vi "Clear Filter Wheel Timeout Flag.vi"(0 "Session Handle in":T1, 11 "error in (no error)":errorcluster) -> (4 "Session Handle out":T1, 6 "Success?":bool, 8 "Error Code":string, 15 "error out":errorcluster)   [LabVIEW 2015, in "PAS.lvclass"]
uses:
  PAS.lvclass
  Typedefs/Session Handle.ctl
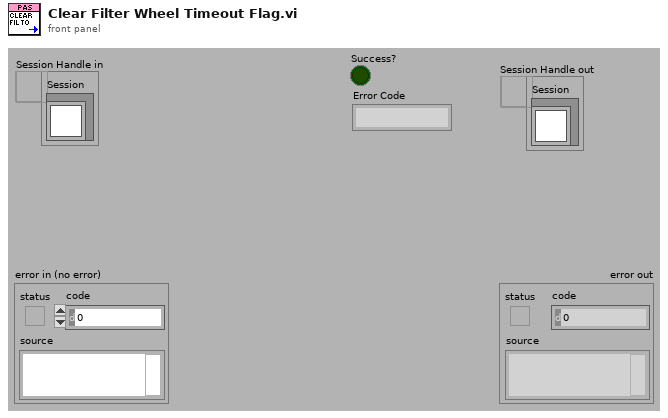
[diagram p1: front panel]
types:
  T1 = typedef "PAS.lvclass/Session Handle.ctl" = refnum<data-value>
  T2 = typedef "XNET Frame CAN.ctl" = cluster{"timestamp":timestamp, "payload":u8[], "identifier":u32, "type":T3, "extended?":bool, "echo?":bool}
  T3 = typedef "XNET Frame Type CAN.ctl" = u8
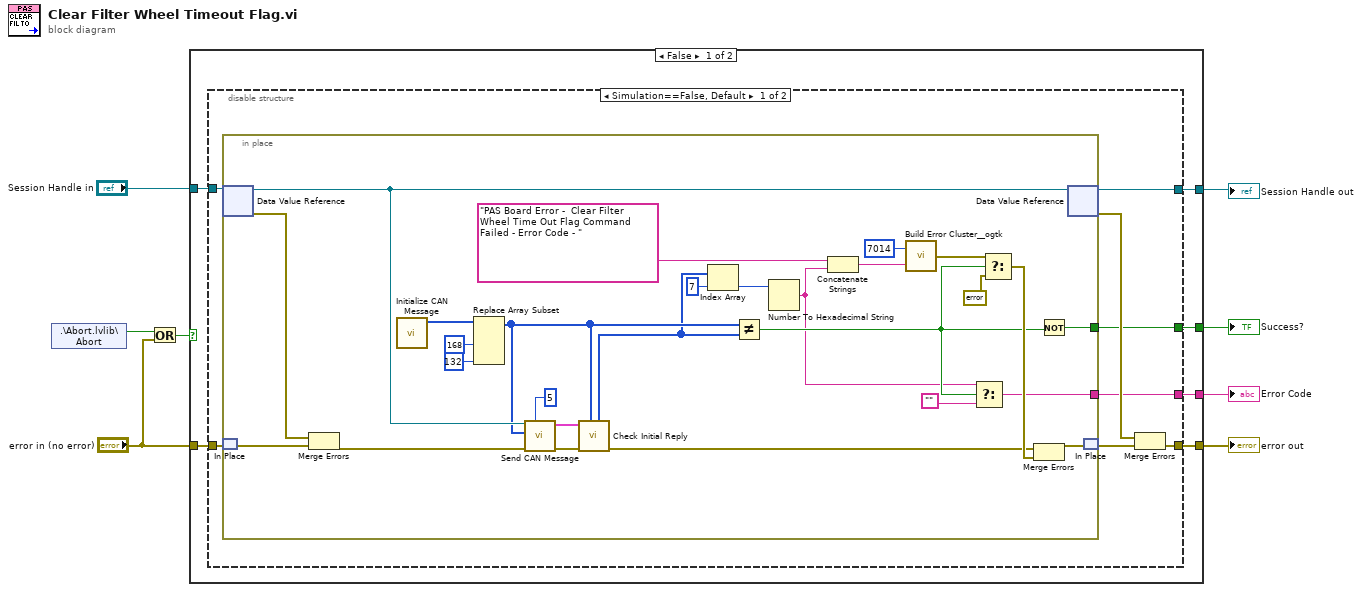
[diagram p0: block diagram]
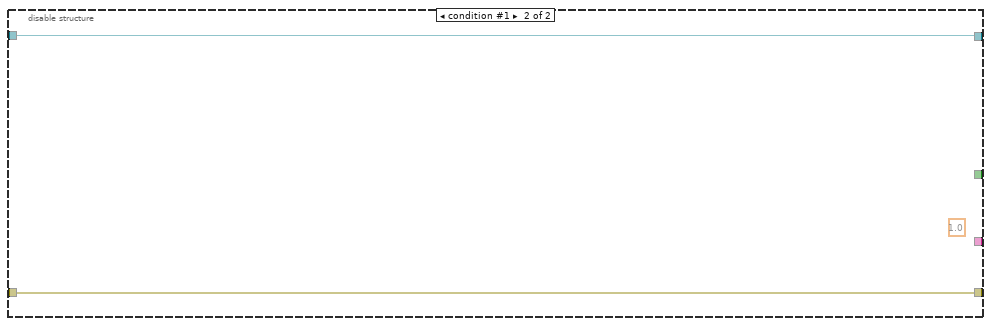
[diagram p2: hidden frame]
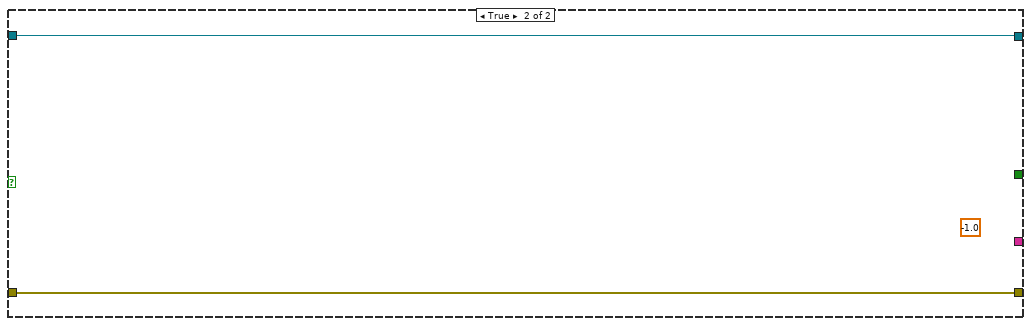
[diagram p3: hidden frame]
diagram:
  n1 = shared-variable ".\\Abort.lvlib\\Abort"() -> (w5:bool)  [unwired: 1 in, 1 out]
  n2 = Or(x=w5, y="error in (no error)") -> (x .or. y?=w3:bool)
  n3 = case shown="False" w3 {
    tunnel: [w14 w53] -> w7
    tunnel: [w13 w52] -> w6
    tunnel: "Session Handle in" -> [w12 w53]
    tunnel: "error in (no error)" -> [w11 w52]
    tunnel: [w10 _] -> w2
    tunnel: [w9 _] -> w1
    frame False {
      n4 = disable-structure shown="Simulation==False, Default" {
        disable-tunnel: [w22 w51] -> w14
        disable-tunnel: [w19 w50] -> w13
        disable-tunnel: w12 -> [w18 w51]
        disable-tunnel: w11 -> [w17 w50]
        disable-tunnel: [w16 _] -> w10
        disable-tunnel: [w15 _] -> w9
        frame condition #0 (active) {
          n5 = in-place {
            in-place-border: [w39] -> w16
            in-place-border: [w25] -> w15
            n6 = in-place-dvr #1(w18) -> (w42:refnum<class "PAS.lvclass">, w46:errorcluster)
            n7 = in-place-match #2(w17) -> (w45:errorcluster)
            n8 = Merge Errors(w46, w45) -> (w41:errorcluster)
            n9 = call "Initialize CAN Message.vi"() -> ("Initial Payload"=w47:u8[])  [unwired: 11 in]
            n10 = Replace Array Subset(array=w47, new element #1=u8 168 ("new element/subarray"), new element #2=u8 132 ("new element/subarray")) -> (w34:u8[])  [unwired: 2 in]
            n11 = call "Send CAN Message.vi"("Number of Retries"=5, "error in (no error)"=w41, "payload"=w34, "Pas In"=w42) -> ("error out"=w24:errorcluster, "Reply"=w43:T2[])  [unwired: 5 in, 1 out]
            n12 = call "Check Initial Reply.vi"("Write Message"=w34, "error in (no error)"=w24, "Reply"=w43) -> ("error out"=w23:errorcluster, "Whole Payload"=w33:u8[])  [unwired: 5 in, 2 out]
            n13 = Index Array(array=w33, index=7) -> (element=w31:u8)
            n14 = Not Equal?(x=w34, y=w33) -> (x != y?=w28:bool)
            n15 = Number To Hexadecimal String(2:w31) -> (0:w27:string)  [unwired: 1 in]
            n16 = Concatenate Strings("PAS Board Error -  Clear Filter Wheel Time Out Flag Command Failed - Error Code - " ("string"), w27) -> (w29:string)
            n17 = call <userlib>:"Build Error Cluster__ogtk.vi"("String to Prepend to source (\"\")"=w29, "code"=7014) -> ("error out"=w38:errorcluster)
            n18 = Select(t=w27, s=w28, f="") -> (s? t:f=w25:string)
            n19 = Select(t=w38, s=w28, f=errorcluster {"status"=FALSE, "code"=0, "source"=""}) -> (s? t:f=w35:errorcluster)
            n20 = Merge Errors(w23, w35) -> (w48:errorcluster)
            n21 = Not(x=w28) -> (.not. x?=w39:bool)
            n22 = in-place-dvr #1(w42) -> (w22:T1, w20:errorcluster)
            n23 = in-place-match #2(w48) -> (w21:errorcluster)
          }
          n24 = Merge Errors(w20, w21) -> (w19:errorcluster)
        }
        frame condition #1 {
          (unwired) 1.0
        }
      }
    }
    frame True {
      (unwired) -1.0
    }
  }
  "Session Handle out" <- w7
  "error out" <- w6
  "Success?" <- w2
  "Error Code" <- w1
